vi "getMessage.vi"(8 "error in (no error)":errorcluster, 11 "IErrorInfo in":refnum<class "IErrorInfo.lvclass">) -> (0 "error out":errorcluster, 2 "ErrorMessage out":string, 3 "IErrorInfo out":refnum<class "IErrorInfo.lvclass">)   [LabVIEW 2022 SP3, in "openDAQ.lvlib" / "IBaseObject.lvlib" / "IErrorInfo.lvlib" / "IErrorInfo.lvclass"]
uses:
  <instrlib>/openDAQ/Public/Classes/IErrorInfo/IErrorInfo.lvclass
  <instrlib>/openDAQ/Public/Classes/IErrorInfo/IErrorInfo.lvclass/IErrorInfo.ctl
  <instrlib>/openDAQ/Binaries/Windows/x86/copendaq32.dll
  <instrlib>/openDAQ/Public/Classes/daqCoreTypes/IString/IString.lvclass
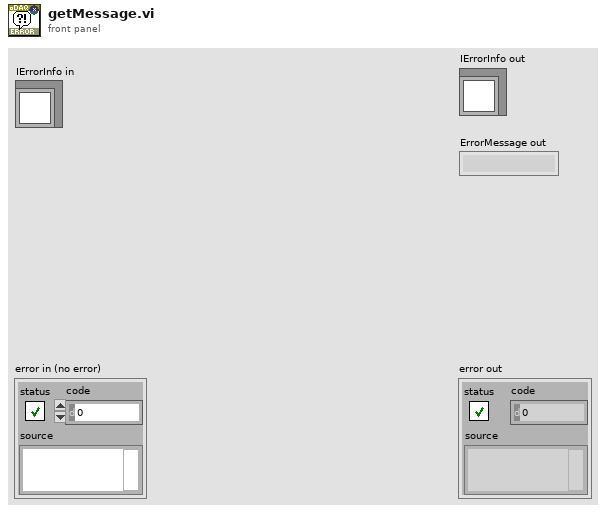
[diagram p1: front panel]
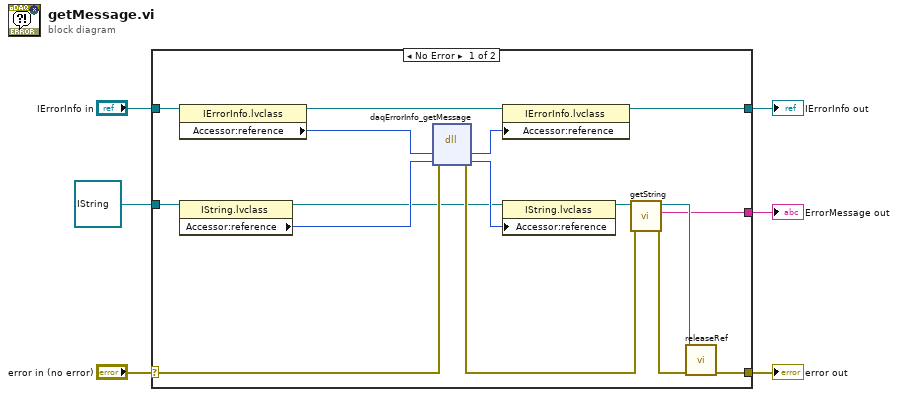
[diagram p0: block diagram]
diagram:
  n1 = case shown="No Error" "error in (no error)" {
    selector: "error in (no error)" -> [w20 w24]
    tunnel: [w14 w24] -> w5
    tunnel: [w19 w23] -> w3
    tunnel: "IErrorInfo in" -> [w8 w23]
    tunnel: refnum<class "IString.lvclass"> refnum ("openDAQ.lvlib:daqCoreTypes.lvlib:IString.lvclass") -> [w10 _]
    tunnel: [w12 _] -> w1
    frame No Error {
      n2 = property class="IErrorInfo.lvclass"(reference=w8) -> (reference out=w7:refnum<class "IErrorInfo.lvclass">, "Accessor:reference"=w22:i64)  [unwired: 1 in, 1 out]
      n3 = property class="IString.lvclass"(reference=w10) -> (reference out=w9:refnum<class "IString.lvclass">, "Accessor:reference"=w21:i64)  [unwired: 1 in, 1 out]
      n4 = dll-call lib="C:/Program Files (x86)/National Instruments/LabVIEW 2022/instr.lib/openDAQ/Binaries/Windows/x86/copendaq*.*" fn="daqErrorInfo_getMessage"(error in=w20, "errorInfo"=w22, "errorMessage"=w21) -> (error out=w16:errorcluster, "errorInfo"=w18:i64, "errorMessage"=w11:i64)  [unwired: 3 in, 1 out]
      n5 = property class="IErrorInfo.lvclass"(reference=w7, "Accessor:reference"=w18) -> (reference out=w19:refnum<class "IErrorInfo.lvclass">)  [unwired: 1 in, 1 out]
      n6 = property class="IString.lvclass"(reference=w9, "Accessor:reference"=w11) -> (reference out=w17:refnum<class "IString.lvclass">)  [unwired: 1 in, 1 out]
      n7 = call <instrlib>:"getString.vi"("error in (no error)"=w16, "IString in"=w17) -> ("error out"=w15:errorcluster, "String out"=w12:string, "IString out"=w13:refnum<class "IString.lvclass">)  [unwired: 7 in]
      n8 = call-dynamic "releaseRef.vi"("error in (no error)"=w15, "IBaseObject in"=w13) -> ("error out"=w14:errorcluster)  [unwired: 9 in]
    }
    frame Error {
    }
  }
  "error out" <- w5
  "IErrorInfo out" <- w3
  "ErrorMessage out" <- w1
